vi "RSNRPZ Close.vi"(8 "error in (no error)":errorcluster, 11 "VISA session":refnum<visa-resource-name>) -> (0 "error out":errorcluster)   [LabVIEW 2014]
doc: "This VI disconnect all channels and close driver session."
uses:
  rsnrpz_32.dll
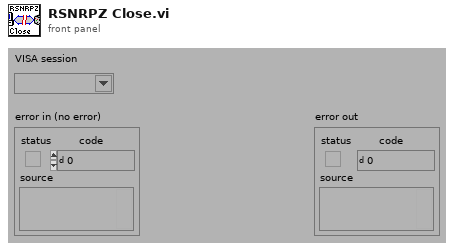
[diagram p1: front panel]
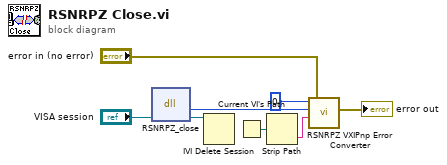
[diagram p0: block diagram]
diagram:
  n1 = dll-call lib="rsnrpz_32.dll" fn="RSNRPZ_close"("Instrument Handle"="VISA session") -> ("Status"=w7:i32)  [unwired: 4 in, 2 out]
  n2 = IVI Delete Session(11:"VISA session") -> ()
  n3 = Current VI's Path() -> (path=w2:path)
  n4 = Strip Path(path=w2) -> (name=w1:string)  [unwired: 1 out]
  n5 = call "RSNRPZ VXIPnp Error Converter.vi"("error in (no error)"="error in (no error)", "name of VI"=w1, "VXIPnp error code"=w7, "VISA session"=i8 0) -> ("error out"=→"error out":errorcluster)  [unwired: 1 out]
